vi "Get CaseFrame Reference By CaseName.vi"(8 "error in (no error)":errorcluster, 10 "CASE":string, 11 "CSM-Helper in":refnum<class "CSM-Helper.lvclass">) -> (0 "error out":errorcluster, 2 "Frame Refs":refnum<vi>, 3 "CSM-Helper out":refnum<class "CSM-Helper.lvclass">)   [LabVIEW 2020, in "CSM-Helper.lvclass"]
uses:
  CSM-Helper.lvclass
  CSM-Helper.lvclass/CSM-Helper.ctl
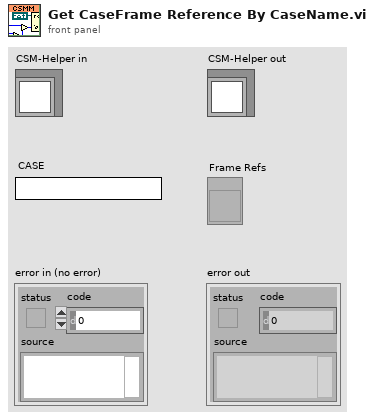
[diagram p1: front panel]
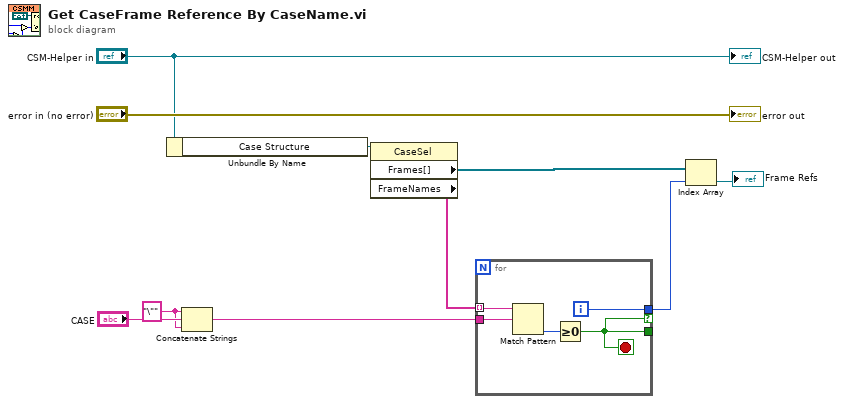
[diagram p0: block diagram]
diagram:
  w4 = "\"" ("string")
  n1 = Unbundle By Name("CSM-Helper in") -> ("Case Structure"=w8:refnum<vi>)
  n2 = Concatenate Strings(w4, "CASE", w4) -> (w5:string)
  n3 = property class="CaseSel"(reference=w8) -> ("Frames[]"=w3:refnum<vi>[], "FrameNames"=w7:string[])  [unwired: 1 in, 2 out]
  n4 = for {
    tunnel: w7 -> [w15] mode=indexing
    tunnel: w5 -> [w14]
    tunnel: [w13] -> w2 if=w11
    tunnel: [w11] -> _
    i -> [w13]
    stop <- w11 stop-if-true
    n5 = Match Pattern(string=w15, regular expression=w14) -> (offset past match=w12:i32)  [unwired: 1 in, 3 out]
    n6 = Greater Or Equal To 0?(x=w12) -> (x >= 0?=w11:bool)
  }
  n7 = Index Array(array=w3, index=w2) -> (element=→"Frame Refs":refnum<vi>)
  "error out" <- "error in (no error)"
  "CSM-Helper out" <- "CSM-Helper in"
